vi "Untitled 1.vi"() -> ()   [LabVIEW 2021]
uses:
  <vilib>/addons/Electrical Power/Basic/NI_EP_Basic.lvlib
  <vilib>/addons/Electrical Power/EV Power Test/Three Phase Power Measurement/Common/Controls/ep_Power Components (Nonfundamental).ctl
  <vilib>/addons/Electrical Power/EV Power Test/Three Phase Power Measurement/Common/NI_EP_Three Phase_Common.lvlib
  <vilib>/addons/Electrical Power/EV Power Test/Three Phase Power Measurement/Common/Controls/ep_Power Components (Fundamental).ctl
  <vilib>/addons/Electrical Power/EV Power Test/Three Phase Power Measurement/Frequency Analysis/NI_EP_Frequency Domain Power Analysis.lvlib
  <vilib>/addons/Electrical Power/EV Power Test/Three Phase Power Measurement/Time Analysis/NI_EP_Time Domain Power Analysis.lvlib
  <vilib>/addons/Electrical Power/EV Power Test/Three Phase Power Measurement/Common/Controls/ep_Power Value (Nonsinusoidal) (1-Phase).ctl
panel:
  out "detected frequency [Hz]":dbl=-1.0 format="%_6g"
  out "nonfundamental powers":T1 {"harmonic distortion power D_H [VAR]" format="%_6g"; "apparent harmonic power S_H [VA]" format="%_6g"; "voltage distortion power D_V [VAR]" format="%_6g"; "active harmonic power P_H [W]" format="%_6g"; "apparent power S_N [VA]" format="%_6g"; "current distortion power D_I [VAR]" format="%_6g"; "harmonic pollution S_N/S1" format="%_6g"}
  out "fundamental powers":T2 {"active power P1 [W]" format="%_6g"; "apparent power S1 [VA]" format="%_6g"; "reactive power Q1 [VAR]" format="%_6g"; "power factor P1/S1" format="%_6g"}
  in  "electrical frequency [Hz]":dbl=-1.0
  out "combined powers":T3
  out "error out":errorcluster
  in  "error in (no error)":errorcluster
  in  "voltage waveform":waveform(dbl)
  in  "current waveform":waveform(dbl)
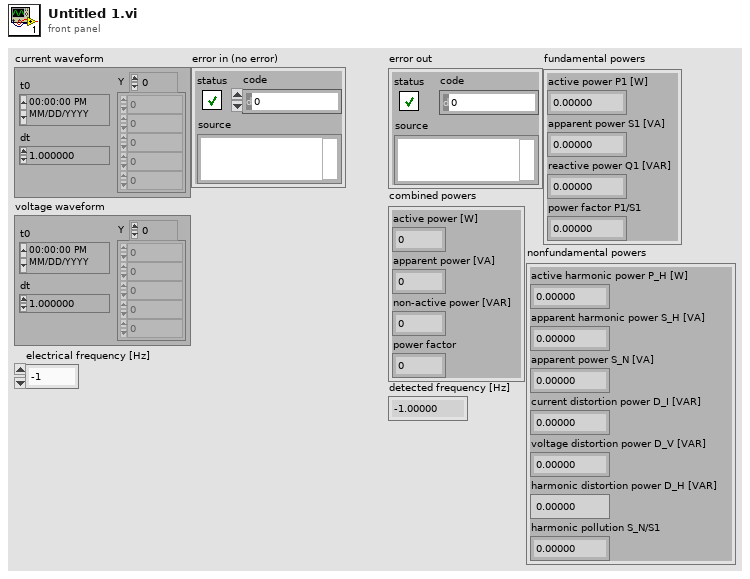
[diagram p1: front panel]
types:
  T1 = typedef "NI_EP_Three Phase_Common.lvlib/ep_Power Components (Nonfundamental).ctl" = cluster{"active harmonic power P_H [W]":dbl, "apparent harmonic power S_H [VA]":dbl, "apparent power S_N [VA]":dbl, "current distortion power D_I [VAR]":dbl, "voltage distortion power D_V [VAR]":dbl, "harmonic distortion power D_H [VAR]":dbl, "harmonic pollution S_N/S1":dbl}
  T2 = typedef "NI_EP_Three Phase_Common.lvlib/ep_Power Components (Fundamental).ctl" = cluster{"active power P1 [W]":dbl, "apparent power S1 [VA]":dbl, "reactive power Q1 [VAR]":dbl, "power factor P1/S1":dbl}
  T3 = typedef "NI_EP_Three Phase_Common.lvlib/ep_Power Value (Nonsinusoidal) (1-Phase).ctl" = cluster{"active power [W]":dbl, "apparent power [VA]":dbl, "non-active power [VAR]":dbl, "power factor":dbl}
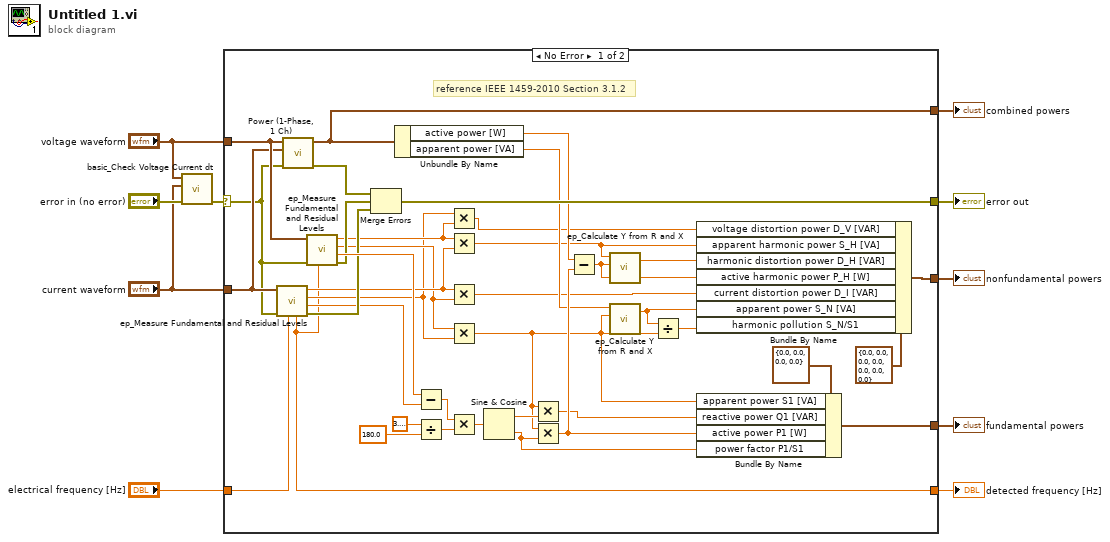
[diagram p0: block diagram]
diagram:
  n1 = call <vilib>:"basic_Check Voltage Current dt.vi"("error in (no error)"="error in (no error)", "current waveform"="current waveform", "voltage waveform"="voltage waveform") -> ("error out"=w7:errorcluster)  [unwired: 8 in]
  n2 = case shown="No Error" w7 {
    selector: w7 -> [w28 w50]
    tunnel: "voltage waveform" -> [w45 _]
    tunnel: "current waveform" -> [w31 _]
    tunnel: [w37 w50] -> w6
    tunnel: [w13 _] -> w5
    tunnel: [w17 _] -> w4
    tunnel: [w14 _] -> w3
    tunnel: "electrical frequency [Hz]" -> [w12 _]
    tunnel: [w11 _] -> w1
    frame No Error {
      # "reference IEEE 1459-2010 Section 3.1.2"
      n3 = call <vilib>:"ep_Measure Fundamental and Residual Levels.vi"("expected frequency (Hz)"=w12, "error in (no error)"=w28, "waveform"=w31) -> ("error out"=w30:errorcluster, "detected phase (deg)"=w29:dbl, "fundamental rms level"=w23:dbl, "residual rms level"=w25:dbl, "detected frequency (Hz)"=w11:dbl)  [unwired: 4 in]
      n4 = call <vilib>:"Power (1-Phase, 1 Ch).vi"("error in (no error)"=w28, "current waveform"=w31, "voltage waveform"=w45) -> ("error out"=w43:errorcluster, "power value"=w13:T3)  [unwired: 7 in]
      n5 = call <vilib>:"ep_Measure Fundamental and Residual Levels.vi"("expected frequency (Hz)"=w11, "error in (no error)"=w28, "waveform"=w45) -> ("error out"=w44:errorcluster, "detected phase (deg)"=w49:dbl, "fundamental rms level"=w24:dbl, "residual rms level"=w26:dbl)  [unwired: 4 in, 1 out]
      n6 = Merge Errors(w43, w44, w30) -> (w37:errorcluster)
      n7 = Unbundle By Name(w13) -> ("active power [W]"=w36:dbl, "apparent power [VA]"=w35:dbl)
      n8 = Subtract(x=w49, y=w29) -> (x-y=w48:dbl)
      n9 = Divide(x=3.141592653589793, y=180.0 ("value")) -> (x/y=w40:dbl)
      n10 = Multiply(x=w23, y=w26) -> (x*y=w21:dbl)
      n11 = Multiply(x=w26, y=w25) -> (x*y=w33:dbl)
      n12 = Multiply(x=w25, y=w24) -> (x*y=w19:dbl)
      n13 = Multiply(x=w24, y=w23) -> (x*y=w27:dbl)
      n14 = Multiply(x=w48, y=w40) -> (x*y=w47:dbl)
      n15 = Sine & Cosine(0:w47) -> (1:w46:dbl, 2:w38:dbl)
      n16 = Multiply(x=w27, y=w46) -> (x*y=w15:dbl)
      n17 = Multiply(x=w27, y=w38) -> (x*y=w39:dbl)
      n18 = Subtract(x=w36, y=w39) -> (x-y=w32:dbl)
      n19 = call <vilib>:"ep_Calculate Y from R and X.vi"("x"=w32, "r"=w33) -> ("y"=w20:dbl)  [unwired: 3 in]
      n20 = call <vilib>:"ep_Calculate Y from R and X.vi"("x"=w27, "r"=w35) -> ("y"=w34:dbl)  [unwired: 3 in]
      n21 = Divide(x=w34, y=w27) -> (x/y=w18:dbl)
      n22 = Bundle By Name(cluster=T1 {"active harmonic power P_H [W]"=0.0, "apparent harmonic power S_H [VA]"=0.0, "apparent power S_N [VA]"=0.0, "current distortion power D_I [VAR]"=0.0, "voltage distortion power D_V [VAR]"=0.0, "harmonic distortion power D_H [VAR]"=0.0, "harmonic pollution S_N/S1"=0.0} ("nonfundamental powers"), "voltage distortion power D_V [VAR]"=w21, "apparent harmonic power S_H [VA]"=w33, "harmonic distortion power D_H [VAR]"=w20, "active harmonic power P_H [W]"=w32, "current distortion power D_I [VAR]"=w19, "apparent power S_N [VA]"=w34, "harmonic pollution S_N/S1"=w18) -> (w17:T1)
      n23 = Bundle By Name(cluster=T2 {"active power P1 [W]"=0.0, "apparent power S1 [VA]"=0.0, "reactive power Q1 [VAR]"=0.0, "power factor P1/S1"=0.0} ("fundamental powers"), "apparent power S1 [VA]"=w27, "reactive power Q1 [VAR]"=w15, "active power P1 [W]"=w39, "power factor P1/S1"=w38) -> (w14:T2)
    }
    frame Error {
    }
  }
  "error out" <- w6
  "combined powers" <- w5
  "fundamental powers" <- w3
  "nonfundamental powers" <- w4
  "detected frequency [Hz]" <- w1
